vi "terminate.vi"(8 "error in (no error)":errorcluster, 11 "MH100301DMC in":refnum<class "StageMH100301DMC.lvclass">) -> (0 "error out":errorcluster, 3 "MH100301DMC out":refnum<class "StageMH100301DMC.lvclass">)   [LabVIEW 2010, in "StageMH100301DMC.lvclass"]
doc: "The dynamic dispatch version of this VI terminates the plug-in object by releasing all of its resources."
uses:
  StageMH100301DMC.lvclass
  StageMH100301DMC.lvclass/StageMH100301DMC.ctl
  StageDL090409Scaffold/StageDL090409Scaffold/StageDL090409Scaffold.lvclass
  common/classes/ErrorController/ErrorController/class_data.vi
  common/classes/ErrorController/ErrorController/ErrorController.lvclass
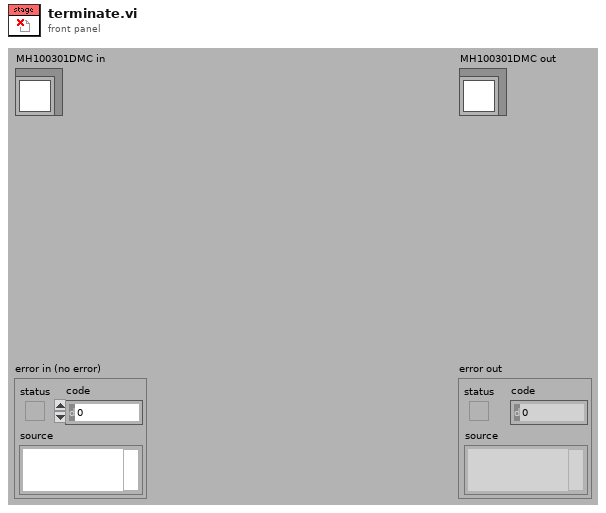
[diagram p1: front panel]
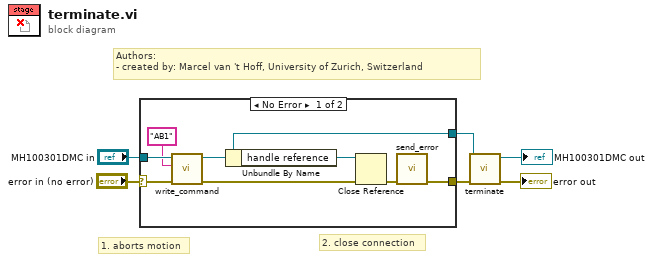
[diagram p0: block diagram]
diagram:
  # "2. close connection"
  # "1. aborts motion"
  # "Authors: \n- created by: Marcel van 't Hoff, University of Zurich, Switzerland"
  n1 = case shown="No Error" "error in (no error)" {
    selector: "error in (no error)" -> [w13 w15]
    tunnel: "MH100301DMC in" -> [w12 w16]
    tunnel: [w10 w16] -> w2
    tunnel: [w14 w15] -> w1
    frame No Error {
      n2 = call-dynamic "write_command.vi"("error in (no error)"=w13, "command (without terminating \"\\n\")"="AB1" ("command (without terminating \"\\n\")"), "MH100301DMC in"=w12) -> ("error out"=w8:errorcluster, "MH100301DMC out"=w10:refnum<class "StageMH100301DMC.lvclass">)  [unwired: 6 in, 1 out]
      n3 = Unbundle By Name(w10) -> ("handle reference"=w9:refnum<k7>)
      n4 = Close Reference(reference=w9, error in (no error)=w8) -> (error out=w7:errorcluster)
      n5 = call "send_error.vi"("error in (no error)"=w7) -> ("error out"=w14:errorcluster)  [unwired: 10 in]
    }
    frame Error {
    }
  }
  n6 = call-parent "terminate.vi"("error in (no error)"=w1, "GenericPlugin in"=w2) -> ("error out"=→"error out":errorcluster, "GenericPlugin out"=→"MH100301DMC out":refnum<class "StageMH100301DMC.lvclass">)  [unwired: 8 out]
